vi "test Create and Look Into Rx Execution Unit Map_NLabelsPerChannel_SDI_Disabled.vi"(8 "error in":errorcluster, 11 "TestCase in":refnum<class "Engine.lvclass">) -> (0 "error out":errorcluster, 3 "TestCase out":refnum<class "Engine.lvclass">)   [LabVIEW 2021, in "Engine.lvclass"]
uses:
  Engine.lvclass
  Shared/RT Hardware Channel Settings.ctl
  Shared/RT Label Settings.ctl
  Shared/Label.ctl
  Shared/RT Parameters.ctl
  Shared/Parameter Definition.ctl
  <vilib>/NI/NI VeriStand Encoding and Decoding/Encoding.ctl
  <vilib>/NI VeriStand/Custom Device API/Custom Device Item Ref.ctl
  Shared/Transfer Type.ctl
  <vilib>/NI VeriStand/Custom Device API/Data Reference.ctl
  <vilib>/addons/_JKI Toolkits/VI Tester/TestCase.llb/TestCase.lvclass
  Engine/Custom Device/Custom Device.lvlib
  <vilib>/NI VeriStand/Custom Device API/Custom Device API.lvlib
  <vilib>/NI/NI VeriStand Encoding and Decoding/Encoding and Decoding.lvlib
  C:/Program Files/National Instruments/LabVIEW 2021/vi.lib/addons/_JKI Toolkits/VI Tester/TestCase.llb/TestCase.lvclass
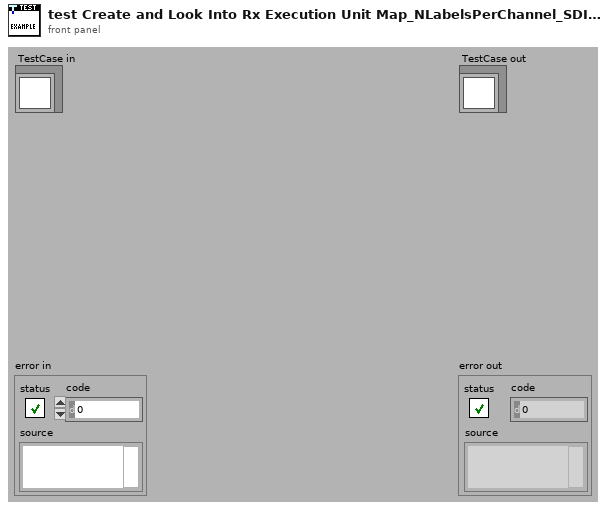
[diagram p1: front panel]
types:
  T1 = typedef "RT Hardware Channel Settings.ctl" = cluster{"channel #":u16, "channel handle":u64, "labels settings for RT":T2[]}
  T2 = typedef "RT Label Settings.ctl" = cluster{"Name":string, "xmlName":string, "label":T3, "transfer period":u32, "SDI_Enabled":bool, "SDI":u8, "parameter driver data":T4, "transfer type":T8, "has timestamp?":bool, "Label Disable/Trigger Channel Reference":T7, "Message Handle":u64, "Initialized?":bool, "Word Initial Raw Value":u32, "Label Timestamp Channel Data Reference":T9, "disabled":bool}
  T3 = typedef "Label.ctl" = u8
  T4 = typedef "RT Parameters.ctl" = cluster{"parameter definitions":T5[], "Tx parameter refs":T7[]}
  T5 = typedef "Parameter Definition.ctl" = cluster{"start index":i32, "size":i32, "encoding":T6, "signed":bool, "scale multiplier":dbl, "scale offset":dbl}
  T6 = typedef "Encoding and Decoding.lvlib/Encoding.ctl" = enum16{"BNR", "BCD", "Discrete"}
  T7 = typedef "Custom Device API.lvlib/Custom Device Item Ref.ctl" = u64
  T8 = typedef "Transfer Type.ctl" = enum16{"Scheduled", "Acyclic", "Block", "Strobe"}
  T9 = typedef "Custom Device API.lvlib/Data Reference.ctl" = i32
  T10 = cluster{"channel index":i32, "label index":i32, "start index":i32, "parameters":i32, "timestamp index":i32}
  T11 = typedef "Map of Identifiers to Indexes.ctl" = map{u32, cluster{"channel index":i32, "label index":i32, "start index":i32, "parameters":i32, "timestamp index":i32}}
  T12 = cluster{"channel index":i32, "label index":i32, "start index":i32, "parameters":i32, "timestamp index":i32}[]
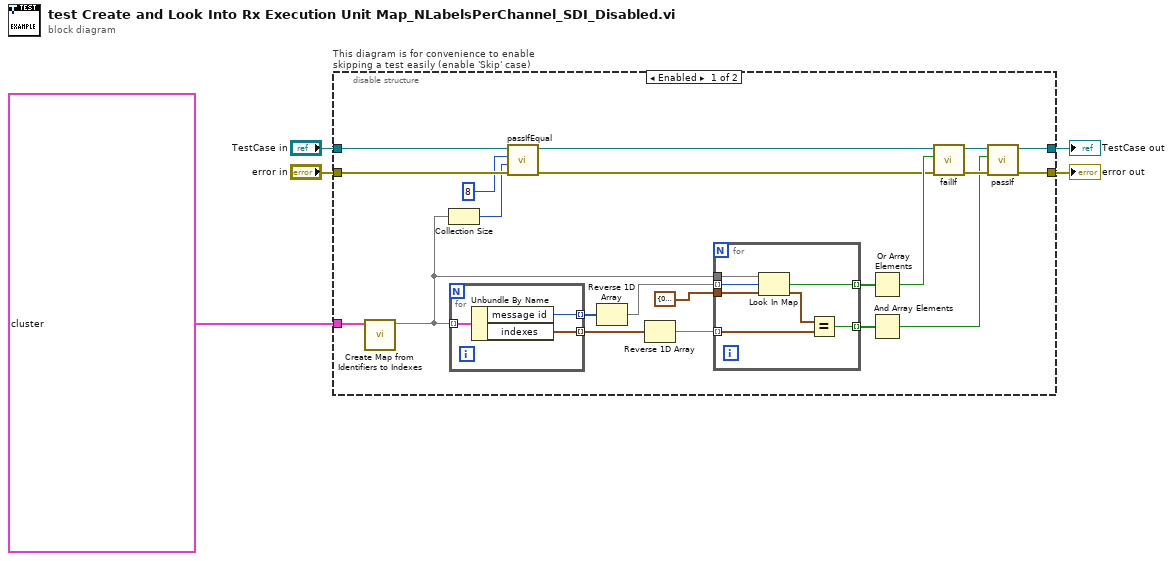
[diagram p0: block diagram]
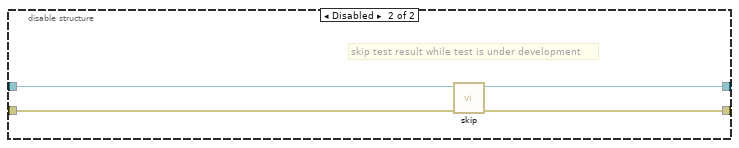
[diagram p2: hidden frame]
diagram:
  n1 = disable-structure "This diagram is for convenience to enable skipping a test easily (enable 'Skip' case)" shown="Enabled" {
    disable-tunnel: "TestCase in" -> [w9 w40]
    disable-tunnel: [w26 w38] -> w2
    disable-tunnel: [w25 w39] -> w4
    disable-tunnel: "error in" -> [w8 w37]
    disable-tunnel: T1[] [{"channel #"=0, "channel handle"=0, "labels settings for RT"=[]}, {"channel #"=1, "channel handle"=0, "labels settings for RT"=[{"Name"="", "xmlName"="", "label"=11, "transfer period"=0, "SDI_Enabled"=FALSE, "SDI"=0, "parameter driver data"={"parameter definitions"=[{"start index"=10, "size"=16, "encoding"=enum."BCD", "signed"=TRUE, "scale multiplier"=1.0, "scale offset"=0.0}], "Tx parameter refs"=[]}, "transfer type"=enum."Scheduled", "has timestamp?"=TRUE, "Label Disable/Trigger Channel Reference"=0, "Message Handle"=0, "Initialized?"=TRUE, "Word Initial Raw Value"=0, "Label Timestamp Channel Data Reference"=0, "disabled"=FALSE}, {"Name"="", "xmlName"="", "label"=55, "transfer period"=0, "SDI_Enabled"=FALSE, "SDI"=0, "parameter driver data"={"parameter definitions"=[{"start index"=15, "size"=11, "encoding"=enum."BNR", "signed"=FALSE, "scale multiplier"=0.0, "scale offset"=0.0}], "Tx parameter refs"=[]}, "transfer type"=enum."Scheduled", "has timestamp?"=FALSE, "Label Disable/Trigger Channel Reference"=0, "Message Handle"=0, "Initialized?"=TRUE, "Word Initial Raw Value"=0, "Label Timestamp Channel Data Reference"=0, "disabled"=FALSE}, {"Name"="", "xmlName"="", "label"=77, "transfer period"=0, "SDI_Enabled"=FALSE, "SDI"=0, "parameter driver data"={"parameter definitions"=[{"start index"=10, "size"=4, "encoding"=enum."BCD", "signed"=FALSE, "scale multiplier"=0.0, "scale offset"=0.0}, {"start index"=14, "size"=2, "encoding"=enum."BNR", "signed"=FALSE, "scale multiplier"=0.0, "scale offset"=0.0}, {"start index"=16, "size"=12, "encoding"=enum."BNR", "signed"=FALSE, "scale multiplier"=0.0, "scale offset"=0.0}], "Tx parameter refs"=[]}, "transfer type"=enum."Scheduled", "has timestamp?"=FALSE, "Label Disable/Trigger Channel Reference"=0, "Message Handle"=0, "Initialized?"=TRUE, "Word Initial Raw Value"=0, "Label Timestamp Channel Data Reference"=0, "disabled"=FALSE}]}, {"channel #"=0, "channel handle"=0, "labels settings for RT"=[]}, {"channel #"=3, "channel handle"=0, "labels settings for RT"=[{"Name"="", "xmlName"="", "label"=33, "transfer period"=0, "SDI_Enabled"=FALSE, "SDI"=0, "parameter driver data"={"parameter definitions"=[{"start index"=10, "size"=19, "encoding"=enum."BNR", "signed"=TRUE, "scale multiplier"=0.0, "scale offset"=0.0}], "Tx parameter refs"=[]}, "transfer type"=enum."Scheduled", "has timestamp?"=FALSE, "Label Disable/Trigger Channel Reference"=0, "Message Handle"=0, "Initialized?"=TRUE, "Word Initial Raw Value"=0, "Label Timestamp Channel Data Reference"=0, "disabled"=FALSE}]}, {"channel #"=0, "channel handle"=0, "labels settings for RT"=[]}, {"channel #"=5, "channel handle"=0, "labels settings for RT"=[{"Name"="", "xmlName"="", "label"=55, "transfer period"=0, "SDI_Enabled"=FALSE, "SDI"=0, "parameter driver data"={"parameter definitions"=[{"start index"=10, "size"=3, "encoding"=enum."BCD", "signed"=FALSE, "scale multiplier"=0.0, "scale offset"=0.0}, {"start index"=13, "size"=4, "encoding"=enum."BCD", "signed"=FALSE, "scale multiplier"=0.0, "scale offset"=0.0}, {"start index"=17, "size"=4, "encoding"=enum."BCD", "signed"=FALSE, "scale multiplier"=0.0, "scale offset"=0.0}, {"start index"=21, "size"=4, "encoding"=enum."BCD", "signed"=FALSE, "scale multiplier"=0.0, "scale offset"=0.0}, {"start index"=25, "size"=4, "encoding"=enum."BCD", "signed"=FALSE, "scale multiplier"=0.0, "scale offset"=0.0}], "Tx parameter refs"=[]}, "transfer type"=enum."Scheduled", "has timestamp?"=FALSE, "Label Disable/Trigger Channel Reference"=0, "Message Handle"=0, "Initialized?"=TRUE, "Word Initial Raw Value"=0, "Label Timestamp Channel Data Reference"=0, "disabled"=FALSE}, {"Name"="", "xmlName"="", "label"=255, "transfer period"=0, "SDI_Enabled"=FALSE, "SDI"=0, "parameter driver data"={"parameter definitions"=[{"start index"=29, "size"=2, "encoding"=enum."BNR", "signed"=FALSE, "scale multiplier"=0.0, "scale offset"=0.0}], "Tx parameter refs"=[]}, "transfer type"=enum."Scheduled", "has timestamp?"=FALSE, "Label Disable/Trigger Channel Reference"=0, "Message Handle"=0, "Initialized?"=TRUE, "Word Initial Raw Value"=0, "Label Timestamp Channel Data Reference"=0, "disabled"=FALSE}]}, {"channel #"=0, "channel handle"=0, "labels settings for RT"=[]}, {"channel #"=0, "channel handle"=0, "labels settings for RT"=[]}, {"channel #"=0, "channel handle"=0, "labels settings for RT"=[]}, {"channel #"=0, "channel handle"=0, "labels settings for RT"=[]}, {"channel #"=0, "channel handle"=0, "labels settings for RT"=[]}, {"channel #"=0, "channel handle"=0, "labels settings for RT"=[]}, {"channel #"=0, "channel handle"=0, "labels settings for RT"=[]}, {"channel #"=0, "channel handle"=0, "labels settings for RT"=[]}, {"channel #"=0, "channel handle"=0, "labels settings for RT"=[]}, {"channel #"=15, "channel handle"=0, "labels settings for RT"=[{"Name"="", "xmlName"="", "label"=155, "transfer period"=0, "SDI_Enabled"=FALSE, "SDI"=0, "parameter driver data"={"parameter definitions"=[{"start index"=10, "size"=1, "encoding"=enum."Discrete", "signed"=FALSE, "scale multiplier"=0.0, "scale offset"=0.0}, {"start index"=11, "size"=1, "encoding"=enum."Discrete", "signed"=FALSE, "scale multiplier"=0.0, "scale offset"=0.0}, {"start index"=12, "size"=1, "encoding"=enum."Discrete", "signed"=FALSE, "scale multiplier"=0.0, "scale offset"=0.0}, {"start index"=13, "size"=1, "encoding"=enum."Discrete", "signed"=FALSE, "scale multiplier"=0.0, "scale offset"=0.0}, {"start index"=14, "size"=1, "encoding"=enum."Discrete", "signed"=FALSE, "scale multiplier"=0.0, "scale offset"=0.0}], "Tx parameter refs"=[]}, "transfer type"=enum."Scheduled", "has timestamp?"=FALSE, "Label Disable/Trigger Channel Reference"=0, "Message Handle"=0, "Initialized?"=TRUE, "Word Initial Raw Value"=0, "Label Timestamp Channel Data Reference"=0, "disabled"=FALSE}]}, {"channel #"=0, "channel handle"=0, "labels settings for RT"=[]}, {"channel #"=0, "channel handle"=0, "labels settings for RT"=[]}, {"channel #"=0, "channel handle"=0, "labels settings for RT"=[]}, {"channel #"=0, "channel handle"=0, "labels settings for RT"=[]}, {"channel #"=0, "channel handle"=0, "labels settings for RT"=[]}, {"channel #"=0, "channel handle"=0, "labels settings for RT"=[]}, {"channel #"=0, "channel handle"=0, "labels settings for RT"=[]}, {"channel #"=0, "channel handle"=0, "labels settings for RT"=[]}, {"channel #"=0, "channel handle"=0, "labels settings for RT"=[]}, {"channel #"=25, "channel handle"=0, "labels settings for RT"=[{"Name"="", "xmlName"="", "label"=255, "transfer period"=0, "SDI_Enabled"=FALSE, "SDI"=0, "parameter driver data"={"parameter definitions"=[{"start index"=0, "size"=0, "encoding"=enum."BNR", "signed"=FALSE, "scale multiplier"=0.0, "scale offset"=0.0}], "Tx parameter refs"=[]}, "transfer type"=enum."Scheduled", "has timestamp?"=FALSE, "Label Disable/Trigger Channel Reference"=0, "Message Handle"=0, "Initialized?"=TRUE, "Word Initial Raw Value"=0, "Label Timestamp Channel Data Reference"=0, "disabled"=FALSE}]}] ("RT hardware channel data") -> [w24 _]
    frame Enabled {
      n2 = call "Create Map from Identifiers to Indexes.vi"("RT hardware channel data"=w24) -> ("map from identifiers to indexes"=w12:T11)  [unwired: 10 in]
      n3 = Collection Size(1:w12) -> (0:w7:i32)
      n4 = for {
        tunnel: w12 -> [w36] mode=indexing
        tunnel: [w35] -> w23 mode=indexing
        tunnel: [w34] -> w22 mode=indexing
        n5 = Unbundle By Name(w36) -> ("message id"=w35:u32, "indexes"=w34:T10)
      }
      n6 = call-dynamic "passIfEqual.vi"("error in (no error)"=w8, "y"=w7, "x"=8 ("size"), "TestCase in"=w9) -> ("error out"=w10:errorcluster, "TestCase out"=w11:refnum<class "Engine.lvclass">)  [unwired: 6 in]
      n7 = Reverse 1D Array(array=w23) -> (reversed array=w21:u32[])
      n8 = Reverse 1D Array(array=w22) -> (reversed array=w15:T12)
      n9 = for {
        tunnel: w12 -> [w33]
        tunnel: w21 -> [w32] mode=indexing
        tunnel: T10 {"channel index"=0, "label index"=0, "start index"=0, "parameters"=0, "timestamp index"=0} ("default value") -> [w31]
        tunnel: [w30] -> w19 mode=indexing
        tunnel: w15 -> [w28] mode=indexing
        tunnel: [w27] -> w14 mode=indexing
        n10 = Look In Map(map=w33, key=w32, default value=w31) -> (key not found?=w30:bool, value=w29:T10)
        n11 = Equal?(x=w29, y=w28) -> (x = y?=w27:bool)
      }
      n12 = Or Array Elements(Boolean array=w19) -> (logical OR=w18:bool)
      n13 = And Array Elements(Boolean array=w14) -> (logical AND=w13:bool)
      n14 = call-dynamic "failIf.vi"("error in (no error)"=w10, "fail"=w18, "TestCase in"=w11) -> ("error out"=w16:errorcluster, "TestCase out"=w17:refnum<class "Engine.lvclass">)  [unwired: 7 in]
      n15 = call-dynamic "passIf.vi"("error in (no error)"=w16, "pass"=w13, "TestCase in"=w17) -> ("error out"=w25:errorcluster, "TestCase out"=w26:refnum<class "Engine.lvclass">)  [unwired: 7 in]
    }
    frame Disabled {
      # "skip test result while test is under development"
      n16 = call <vilib>:"skip.vi"("error in (no error)"=w37, "TestCase in"=w40) -> ("error out"=w39:errorcluster, "TestCase out"=w38:refnum<class "Engine.lvclass">)  [unwired: 8 in]
    }
  }
  "error out" <- w4
  "TestCase out" <- w2
